vi "Part 2.vi"(11 "Input":string) -> (3 "Output":i64)   [LabVIEW 2021]
uses:
  142248e0-e750-4ede-a8fc-2e630f83094c.vi
  <userlib>/_OpenG.lib/string/string.llb/Convert EOLs (String)__ogtk.vi
  <vilib>/Comparison/Less/Less Functor/Less Functor.lvclass
panel:
  out "Minimum directory size":i64
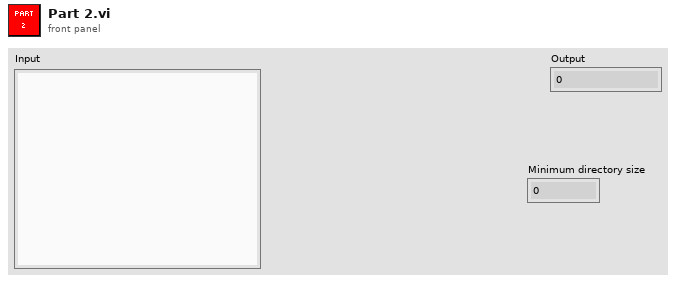
[diagram p1: front panel]
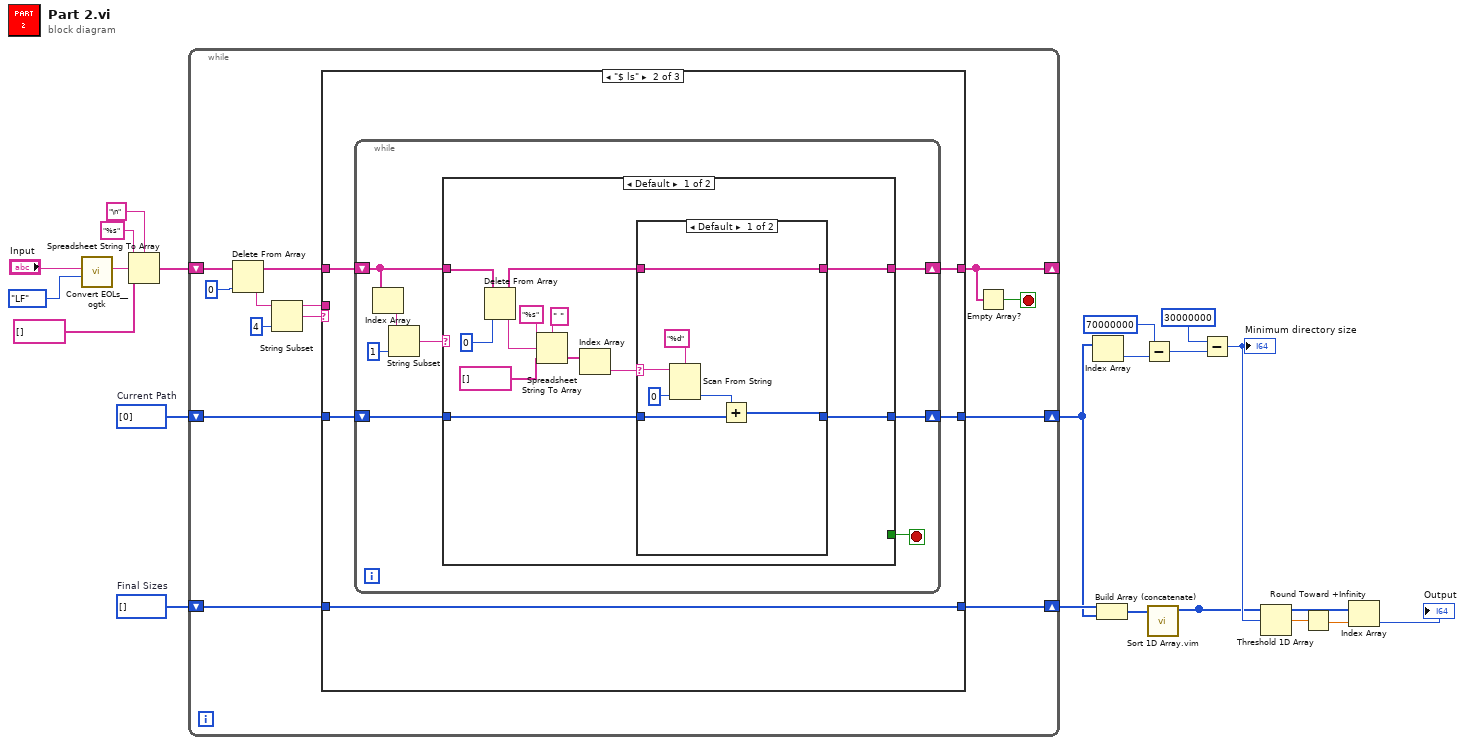
[diagram p0: block diagram]
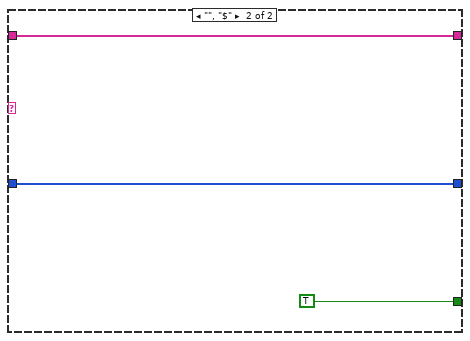
[diagram p4: hidden frame]
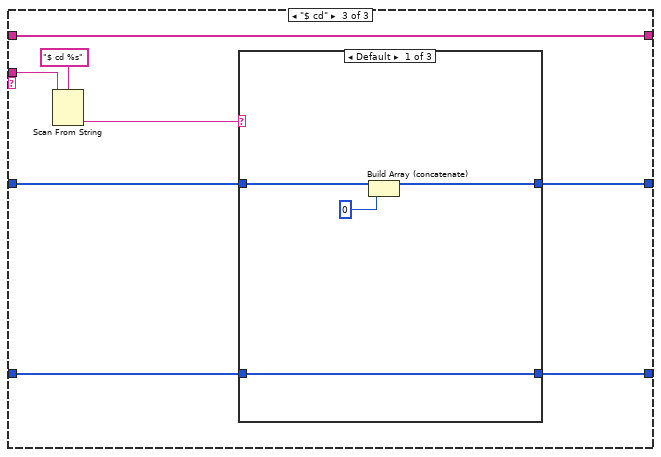
[diagram p5: hidden frame]
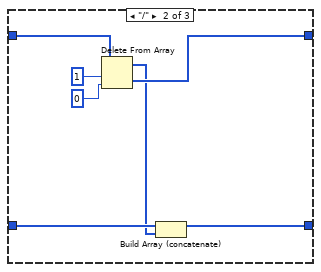
[diagram p6: hidden frame]
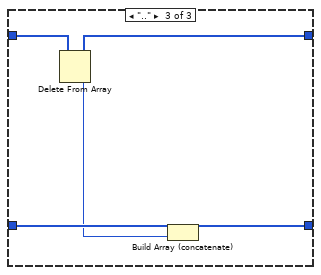
[diagram p7: hidden frame]
diagram:
  w14 = i64[] []  # Final Sizes
  w15 = i64[] [0]  # Current Path
  n1 = call-poly <userlib>:"Convert EOLs__ogtk.vi"("Convert to:"=enum16{"CR", "LF", "CRLF"}."LF", "String in"="Input") -> ("String out"=w20:string)  [unwired: 9 in]
  n2 = Spreadsheet String To Array(delimiter (Tab)="\n", format string="%s", spreadsheet string=w20, array type (2D Dbl)=string[] []) -> (array=w16:string[])
  n3 = while {
    shift-right: [w28] -> _
    shift-left: w16 -> [w33]
    shift-right: [w24] -> w11
    shift-left: w15 -> [w26]
    shift-right: [w22] -> w13
    shift-left: w14 -> [w23]
    stop <- w27 stop-if-true
    n4 = Delete From Array(array=w33, index=0) -> (deleted portion=w25:string, array with subset deleted=w29:string[])  [unwired: 1 in]
    n5 = String Subset(string=w25, length (rest)=4 ("length (rest)")) -> (substring=w30:string)  [unwired: 1 in]
    n6 = case shown="\"$ ls\"" w30 {
      tunnel: w29 -> [w36 w40 w81]
      tunnel: [w36 w39 w81] -> w28
      tunnel: w26 -> [w35 w38 w77]
      tunnel: w25 -> [_ _ w80]
      tunnel: [w35 w37 w76] -> w24
      tunnel: w23 -> [w34 w41 w75]
      tunnel: [w34 w41 w74] -> w22
      frame Default {
      }
      frame "$ ls" {
        n7 = while {
          shift-right: [w45] -> w39
          shift-left: w40 -> [w46]
          shift-right: [w43] -> w37
          shift-left: w38 -> [w44]
          stop <- w42 stop-if-true
          n8 = Index Array(array=w46) -> (element=w49:string)  [unwired: 1 in]
          n9 = String Subset(string=w49, length (rest)=1 ("length (rest)")) -> (substring=w47:string)  [unwired: 1 in]
          n10 = case shown="Default" w47 {
            tunnel: w46 -> [w60 w73]
            tunnel: [w53 w73] -> w45
            tunnel: w44 -> [w51 w72]
            tunnel: [w52 w72] -> w43
            tunnel: [_ TRUE] -> w42
            frame Default {
              n11 = Delete From Array(array=w60, index=0) -> (deleted portion=w59:string, array with subset deleted=w54:string[])  [unwired: 1 in]
              n12 = Spreadsheet String To Array(delimiter (Tab)=" ", format string="%s", spreadsheet string=w59, array type (2D Dbl)=string[] []) -> (array=w56:string[])
              n13 = Index Array(array=w56) -> (element=w55:string)  [unwired: 1 in]
              n14 = case shown="Default" w55 {
                selector: w55 -> [w68 _]
                tunnel: w54 -> [w64 w70]
                tunnel: [w64 w70] -> w53
                tunnel: [w63 w69] -> w52
                tunnel: w51 -> [w66 w69]
                frame Default {
                  n15 = Scan From String(format string="%d", input string=w68, default 1=i64 0) -> (output 1=w65:i64)  [unwired: 2 in, 3 out]
                  n16 = Add(x=w65, y=w66) -> (x+y=w63:i64[])
                }
                frame "dir" {
                }
              }
            }
            frame "", "$" {
            }
          }
        }
      }
      frame "$ cd" {
        n17 = Scan From String(format string="$ cd %s", input string=w80) -> (output 1=w78:string)  [unwired: 3 in, 3 out]
        n18 = case shown="Default" w78 {
          tunnel: w77 -> [w84 w89 w96]
          tunnel: [w82 w90 w97] -> w76
          tunnel: w75 -> [w85 w88 w95]
          tunnel: [w85 w86 w93] -> w74
          frame Default {
            n19 = Build Array (concatenate)(w84, i64 0) -> (w82:i64[])
          }
          frame "/" {
            n20 = Delete From Array(array=w89, length=1, index=0) -> (deleted portion=w90:i64[], array with subset deleted=w87:i64[])
            n21 = Build Array (concatenate)(w88, w87) -> (w86:i64[])
          }
          frame ".." {
            n22 = Delete From Array(array=w96) -> (deleted portion=w94:i64, array with subset deleted=w97:i64[])  [unwired: 2 in]
            n23 = Build Array (concatenate)(w95, w94) -> (w93:i64[])
          }
        }
      }
    }
    n24 = Empty Array?(array=w28) -> (empty?=w27:bool)
  }
  n25 = Index Array(array=w11) -> (element=w10:i64)  [unwired: 1 in]
  n26 = Build Array (concatenate)(w13, w11) -> (w6:i64[])
  n27 = Subtract(x=i64 70000000, y=w10) -> (x-y=w8:i64)
  n28 = call "Sort 1D Array.vim"("unsorted array"=w6) -> ("sorted array"=w2:i64[])  [unwired: 10 in]
  n29 = Subtract(x=i64 30000000, y=w8) -> (x-y=w5:i64)
  "Minimum directory size" <- w5
  n30 = Threshold 1D Array(2:w5, 3:w2) -> (0:w4:dbl)  [unwired: 1 in]
  n31 = Round Toward +Infinity(x=w4) -> (ceil(x): smallest int >= x=w3:dbl)
  n32 = Index Array(array=w2, index=w3) -> (element=→"Output":i64)
